vi "aryscan set.vi"(7 "fly back step #":dbl, 8 "error in (no error)":errorcluster {"code" format="%.0x"}, 10 "p Cluster":T3={"exposure time"=3.8e-05, "frame #"=20, "x#"=0.0, "y#"=0.0, "x step size"=0.0, "y step size"=0.0, "buffer page size"=0.0} {"buffer page size" min=0.0 max=2044.0 step=4.0; "y#" min=0.0 max=2044.0 step=4.0; "x#" min=0.0 max=2044.0 step=4.0; "y step size" min=0.0 max=2044.0 step=4.0; "x step size" min=0.0 max=2044.0 step=4.0; "frame #" min=4 max=2048 step=4; "exposure time" min=0.0 max=10.0 step=0.1}, 11 "Camera handle in":u32) -> (0 "error out":errorcluster, 2 "buffer array":T2[](array[typedef]), 3 "Handle out":u32, 4 "actual exposure time":dbl)   [LabVIEW 2015]
uses:
  Control 1.ctl
  <vilib>/vision/Image Controls.llb/IMAQ Image.ctl
panel:
  out "Function List":T1(array[cluster])
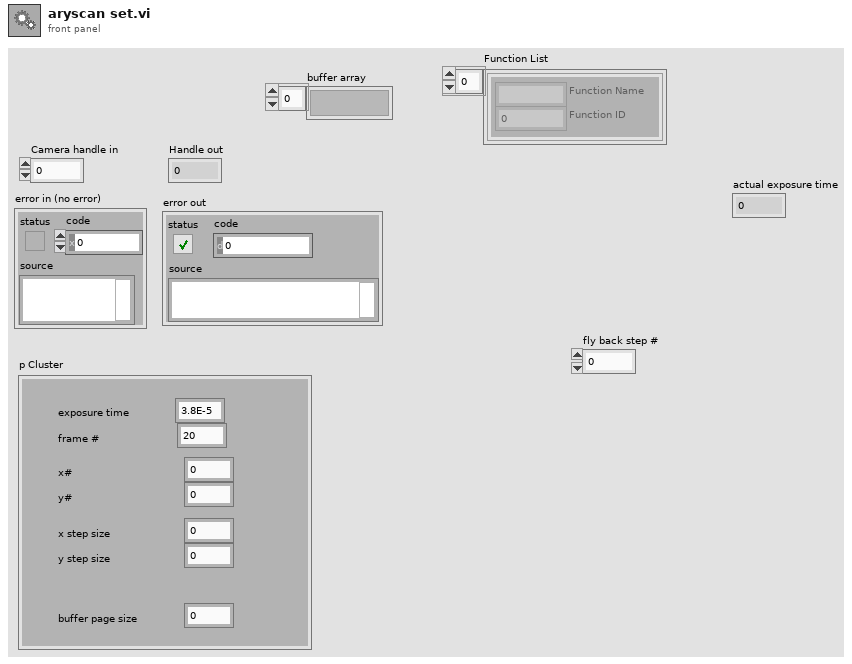
[diagram p1: front panel]
types:
  T1 = cluster{"Function Name":string, "Function ID":u32}[]
  T2 = typedef "IMAQ Image.ctl" = refnum<image>
  T3 = typedef "Control 1.ctl" = cluster{"exposure time":dbl, "frame #":u16, "x#":dbl, "y#":dbl, "x step size":dbl, "y step size":dbl, "buffer page size":dbl}
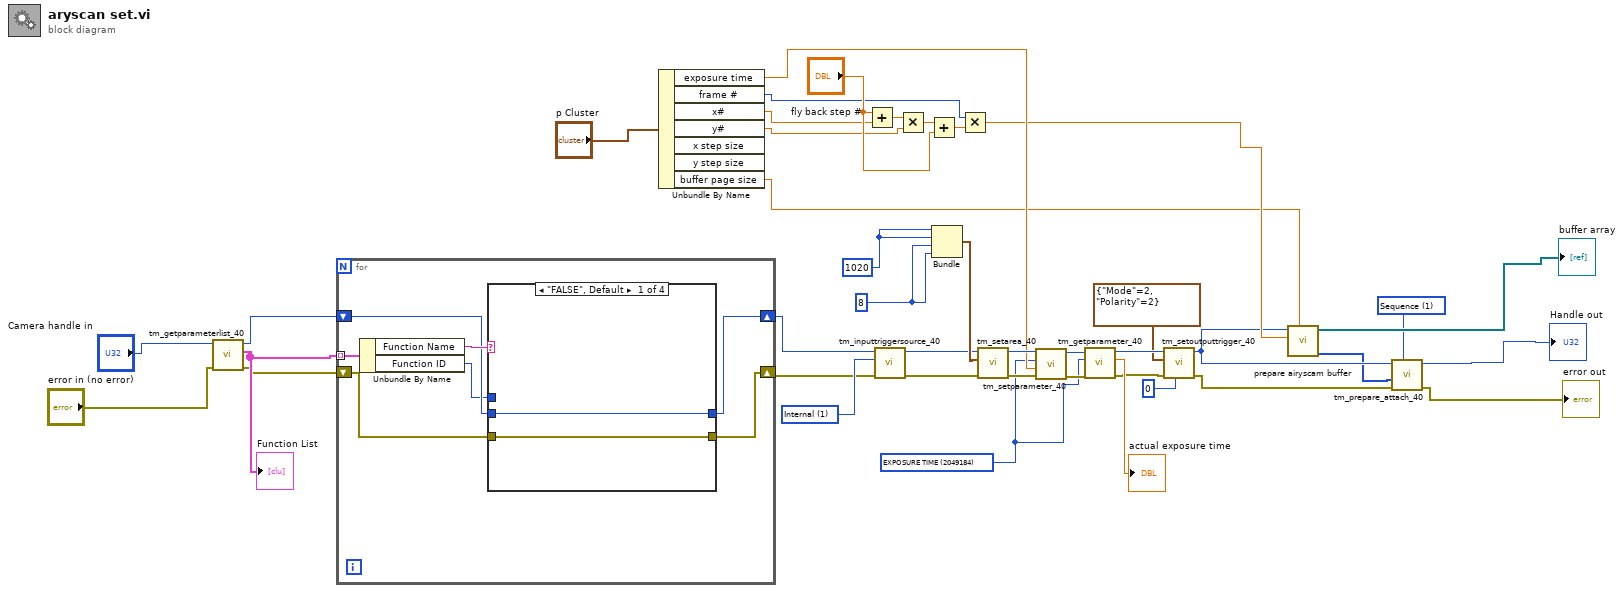
[diagram p0: block diagram]
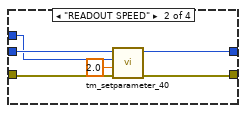
[diagram p2: hidden frame]
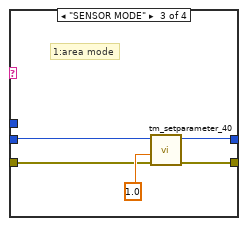
[diagram p3: hidden frame]
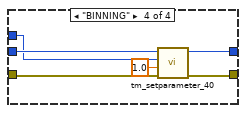
[diagram p4: hidden frame]
diagram:
  w1 = 1 items=["Snap", "Sequence"] ("Capture mode")
  w27 = 1 items=["Internal"=1, "External"=2, "Software"=3, "Master Pulse"=4] ("Source")
  w31 = u32 2049184 items=["SENSOR MODE"=4212128, "READOUT SPEED"=4211872, "READOUT DIRECTION"=4211904, "TRIGGER GLOBAL EXPOSURE"=2049680, "TRIGGER DELAY"=1066480, "INTERNAL TRIGGER HANDLING"=1066496, "SYNC READOUT SYSTEM BLANK"=1066528, "SENSOR TEMPERATURE"=2115232, "SENSOR COOLER STATUS"=2115280, "EXPOSURE TIME"=2049184, "DEFECT CORRECT MODE"=4670368, "BINNING"=4215968, "INTERNAL LINE SPEED"=4226000, "INTERNAL LINE INTERVAL"=4226016, "NUMBER OF OUTPUT TRIGGER CONNECTOR"=1852320, "OUTPUT TRIGGER SOURCE[0]"=1852576, "OUTPUT TRIGGER SOURCE[1]"=1852832, "OUTPUT TRIGGER SOURCE[2]"=1853088, "OUTPUT TRIGGER POLARITY[0]"=1852592, "OUTPUT TRIGGER POLARITY[1]"=1852848, "OUTPUT TRIGGER POLARITY[2]"=1853104, "OUTPUT TRIGGER ACTIVE[0]"=1852608, "OUTPUT TRIGGER ACTIVE[1]"=1852864, "OUTPUT TRIGGER ACTIVE[2]"=1853120, "OUTPUT TRIGGER DELAY[0]"=1852624, "OUTPUT TRIGGER DELAY[1]"=1852880, "OUTPUT TRIGGER DELAY[2]"=1853136, "OUTPUT TRIGGER PERIOD[0]"=1852640, "OUTPUT TRIGGER PERIOD[1]"=1852896, "OUTPUT TRIGGER PERIOD[2]"=1853152, "OUTPUT TRIGGER KIND[0]"=1852656, "OUTPUT TRIGGER KIND[1]"=1852912, "OUTPUT TRIGGER KIND[2]"=1853168, "OUTPUT TRIGGER BASE SENSOR[0]"=1852672, "OUTPUT TRIGGER BASE SENSOR[1]"=1852928, "OUTPUT TRIGGER BASE SENSOR[2]"=1853184, "OUTPUT TRIGGER PRE HSYNC COUNT"=1852704] ("Parameter")
  w38 = 1020
  w3 = 8
  n1 = call <userlib>:"tm_getparameterlist_40.vi"("error in (no error)"="error in (no error)", "Handle in"="Camera handle in") -> ("error out"=w10:errorcluster, "Function List"=w11:T1, "Handle out"=w9:u32)  [unwired: 7 in]
  "Function List" <- w11
  n2 = for {
    tunnel: w11 -> [w48] mode=indexing
    shift-right: [w45] -> w8
    shift-left: w9 -> [w43]
    shift-right: [w44] -> w7
    shift-left: w10 -> [w46]
    n3 = Unbundle By Name(w48) -> ("Function Name"=w47:string, "Function ID"=w42:u32)
    n4 = case shown="\"FALSE\", Default" w47 {
      tunnel: w43 -> [w49 w53 w60 w67]
      tunnel: [w49 w54 w57 w64] -> w45
      tunnel: [w50 w55 w58 w65] -> w44
      tunnel: w46 -> [w50 w56 w59 w66]
      tunnel: w42 -> [_ w52 _ w63]
      frame "FALSE", Default {
      }
      frame "READOUT SPEED" {
        n5 = call <userlib>:"tm_setparameter_40.vi"("error in (no error)"=w56, "Value in"=2.0, "Parameter"=w52, "Handle in"=w53) -> ("error out"=w55:errorcluster, "Handle out"=w54:u32)  [unwired: 6 in]
      }
      frame "SENSOR MODE" {
        # "1:area mode"
        n6 = call <userlib>:"tm_setparameter_40.vi"("error in (no error)"=w59, "Value in"=1.0, "Handle in"=w60) -> ("error out"=w58:errorcluster, "Handle out"=w57:u32)  [unwired: 7 in]
      }
      frame "BINNING" {
        n7 = call <userlib>:"tm_setparameter_40.vi"("error in (no error)"=w66, "Value in"=1.0, "Parameter"=w63, "Handle in"=w67) -> ("error out"=w65:errorcluster, "Handle out"=w64:u32)  [unwired: 6 in]
      }
    }
  }
  n8 = Unbundle By Name("p Cluster") -> ("exposure time"=w32:dbl, "frame #"=w4:u16, "x#"=w17:dbl, "y#"=w16:dbl, "buffer page size"=w25:dbl)  [unwired: 2 out]
  n9 = Add(x="fly back step #", y=w17) -> (x+y=w21:dbl)
  n10 = call <userlib>:"tm_inputtriggersource_40.vi"("error in (no error)"=w7, "Source"=w27, "Handle in"=w8) -> ("error out"=w28:errorcluster, "Handle out"=w29:u32)  [unwired: 7 in]
  n11 = Multiply(x=w21, y=w16) -> (x*y=w20:dbl)
  n12 = Add(x=w20, y="fly back step #") -> (x+y=w18:dbl)
  n13 = Bundle(w38, w38, w3, w3) -> (w37:cluster{i32, i32, i32, i32})  [unwired: 1 in]
  n14 = Multiply(x=w4, y=w18) -> (x*y=w26:dbl)
  n15 = call <userlib>:"tm_setarea_40.vi"("error in (no error)"=w28, "Sub Region"=w37, "Handle in"=w29) -> ("error out"=w36:errorcluster, "Handle out"=w35:u32)  [unwired: 7 in]
  n16 = call <userlib>:"tm_setparameter_40.vi"("error in (no error)"=w36, "Value in"=w32, "Parameter"=w31, "Handle in"=w35) -> ("error out"=w34:errorcluster, "Handle out"=w33:u32)  [unwired: 6 in]
  n17 = call <userlib>:"tm_getparameter_40.vi"("error in (no error)"=w34, "Parameter"=w31, "Handle in"=w33) -> ("error out"=w6:errorcluster, "Value out"=→"actual exposure time":dbl, "Handle out"=w15:u32)  [unwired: 6 in]
  n18 = call <userlib>:"tm_setoutputtrigger_40.vi"("Port"=0, "error in (no error)"=w6, "Type"=cluster{"Mode":u32, "Polarity":u32} {"Mode"=2, "Polarity"=2}, "Handle in"=w15) -> ("error out"=w5:errorcluster, "Handle out"=w14:u32)  [unwired: 6 in]
  n19 = call "prepare airyscam buffer.vi"("buffer page size"=w25, "frames"=w26, "Camera handle in"=w14) -> ("buffer pointers"=w2:u64[], "buffer array"=→"buffer array":T2[])  [unwired: 7 in]
  n20 = call <userlib>:"tm_prepare_attach_40.vi"("error in (no error)"=w5, "buffers"=w2, "Capture mode"=w1, "Handle in"=w14) -> ("error out"=→"error out":errorcluster, "Handle out"=→"Handle out":u32)  [unwired: 6 in]
